vi "Uninit.vi"(2 "Container State":T1, 3 "Display State":T2={"WebView2 Ref"=refnum, "event callback refnum"=refnum, "Events"={"Navigation Complete Event"=refnum, "Source Changed Event"=refnum, "Document Title Changed Event"=refnum, "Status Bar Text Changed"=refnum, "Web Message Received"=refnum, "Window Close Requested"=refnum}, "Paths"={"Webview2 Native"=path "C:/Users/kleins/Desktop/webview2/microsoft.web.webview2.1.0.1370.28/build/native", "Edge Application"=path "", "User Data"=path ""}}) -> ()   [LabVIEW 2020, in "WebView2 Control.xctl"]
uses:
  WebView2 Control.xctl
  State.ctl
  C:/Users/kleins/Desktop/webview2/microsoft.web.webview2.1.0.1370.28/lib/net45/Microsoft.Web.WebView2.WinForms.dll
  microsoft.web.webview2.1.0.1370.28/lib/net45/Microsoft.Web.WebView2.WinForms.dll
  Paths.ctl
  <vilib>/_xctls/Container State.ctl
  <vilib>/_xctls/XControlSupport.lvlib
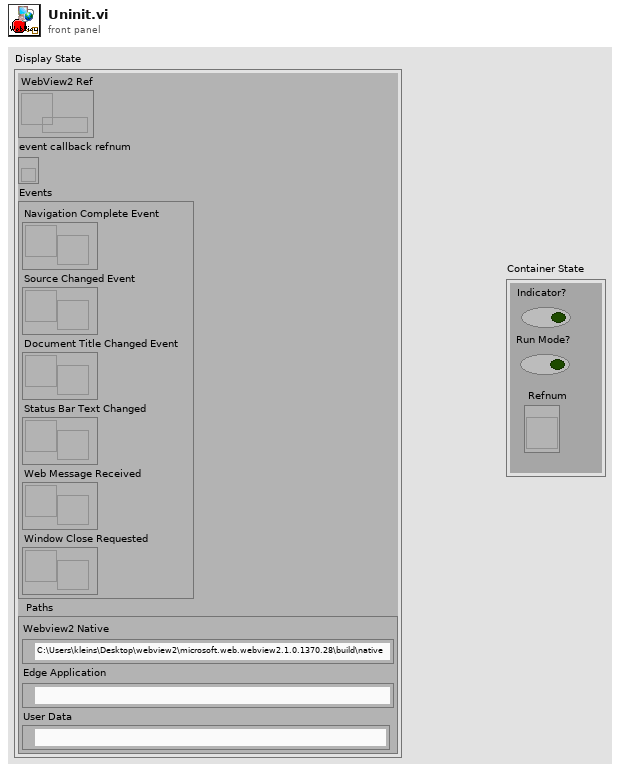
[diagram p1: front panel]
types:
  T1 = typedef "XControlSupport.lvlib/Container State.ctl" = cluster{"Indicator?":bool, "Run Mode?":bool, " Refnum":refnum<vi>}
  T2 = typedef "WebView2 Control.xctl/State.ctl" = cluster{"WebView2 Ref":refnum<data-value>, "event callback refnum":refnum<k27>, "Events":cluster{"Navigation Complete Event":refnum<user-event>, "Source Changed Event":refnum<user-event>, "Document Title Changed Event":refnum<user-event>, "Status Bar Text Changed":refnum<user-event>, "Web Message Received":refnum<user-event>, "Window Close Requested":refnum<user-event>}, "Paths":T3}
  T3 = typedef "WebView2 Control.xctl/Paths.ctl" = cluster{"Webview2 Native":path, "Edge Application":path, "User Data":path}
  T4 = cluster{"Navigation Complete Event":refnum<user-event>, "Source Changed Event":refnum<user-event>, "Document Title Changed Event":refnum<user-event>, "Status Bar Text Changed":refnum<user-event>, "Web Message Received":refnum<user-event>, "Window Close Requested":refnum<user-event>}
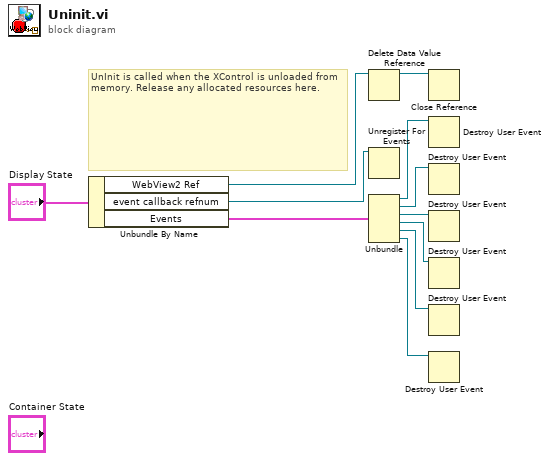
[diagram p0: block diagram]
diagram:
  # "UnInit is called when the XControl is unloaded from memory. Release any allocated resources here."
  n1 = Unbundle By Name("Display State") -> ("WebView2 Ref"=w10:refnum<data-value>, "event callback refnum"=w9:refnum<k27>, "Events"=w8:T4)
  n2 = Delete Data Value Reference(data value reference=w10) -> (data value=w1:refnum<k24>)  [unwired: 1 in, 1 out]
  n3 = Unregister For Events(event registration refnum=w9) -> ()  [unwired: 1 in, 1 out]
  n4 = Unbundle(w8) -> ("Navigation Complete Event"=w7:refnum<user-event>, "Source Changed Event"=w6:refnum<user-event>, "Document Title Changed Event"=w5:refnum<user-event>, "Status Bar Text Changed"=w4:refnum<user-event>, "Web Message Received"=w3:refnum<user-event>, "Window Close Requested"=w2:refnum<user-event>)
  n5 = Close Reference(reference=w1) -> ()  [unwired: 1 in, 1 out]
  n6 = Destroy User Event(user event=w7) -> ()  [unwired: 1 in, 1 out]
  n7 = Destroy User Event(user event=w6) -> ()  [unwired: 1 in, 1 out]
  n8 = Destroy User Event(user event=w5) -> ()  [unwired: 1 in, 1 out]
  n9 = Destroy User Event(user event=w4) -> ()  [unwired: 1 in, 1 out]
  n10 = Destroy User Event(user event=w3) -> ()  [unwired: 1 in, 1 out]
  n11 = Destroy User Event(user event=w2) -> ()  [unwired: 1 in, 1 out]
